vi "DAQ_E_mIO_DIO.port list.vi"(10 "portList":tag="Dev1/port0") -> (2 "nOfBits":i32)   [LabVIEW 2014, in "DAQ_E_mIO_DIO.lvlib"]
doc: "Calculates the numer of used bits from a port list."
uses:
  DAQ_E_mIO_DIO.lvlib
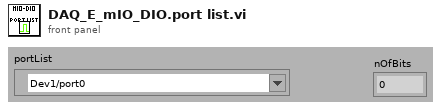
[diagram p1: front panel]
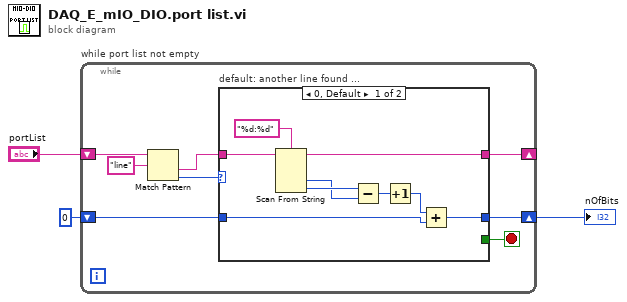
[diagram p0: block diagram]
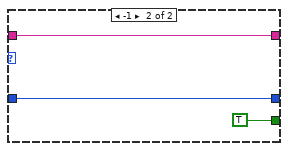
[diagram p2: hidden frame]
diagram:
  n1 = while "while port list not empty" {
    shift-right: [w8] -> w1
    shift-left: 0 -> [w7]
    shift-right: [w6] -> _
    shift-left: "portList" -> [w10]
    stop <- w4 stop-if-true
    n2 = Match Pattern(string=w10, regular expression="line") -> (after substring=w9:string, offset past match=w5:i32)  [unwired: 1 in, 2 out]
    n3 = case "default: another line found ..." shown="0, Default" w5 {
      tunnel: w9 -> [w19 w23]
      tunnel: [w14 w22] -> w8
      tunnel: w7 -> [w13 w22]
      tunnel: [w12 w23] -> w6
      tunnel: [_ TRUE] -> w4
      frame 0, Default {
        n4 = Scan From String(format string="%d:%d", input string=w19) -> (remaining string=w12:string, output 1=w16:i32, output 2=w17:i32)  [unwired: 4 in, 2 out]
        n5 = Subtract(x=w17, y=w16) -> (x-y=w20:i32)
        n6 = Increment(x=w20) -> (x+1=w15:i32)
        n7 = Add(x=w15, y=w13) -> (x+y=w14:i32)
      }
      frame -1 {
      }
    }
  }
  "nOfBits" <- w1
